vi "(SubVI)Serial_User Code Verification.vi"(8 "에러 입력(에러 없음)":errorcluster, 10 "Data to Write":u8[](array[numeric]), 11 "Read Data":u8[](array[numeric])) -> (0 "에러 출력":errorcluster, 3 "Read Data":u8[](array[numeric]))   [LabVIEW 2020]
panel:
  # "(SubVI)Serial_User Code Verification.vi By hspark\n\nDescription : 시리얼 통신 Write-Read 동작 시 프로토콜 중 Header(6Byte) 다음 2Byte에 대해 검증하는 VI\n                   쓰기한 데이터와 읽기한 데이터가 같은 경우 pass. 다를 경우 에러 발생시킴\n\nInput : \n1. Read Data : 시리얼 통신으로 읽은 데이터 입력\n2. Data to Write : 시리얼 통신으로 쓴 데이터 입력\n\nOutput : \n1. Read Data : Read Data 입력 중 검증한 2Byte를 제외한 나머지 데이터 출력\n\nLabVIEW Version : 2020 SP1 이상\n\nNote : 에러 발생 시 에러 코드는 부여하지 않음. 필요 시 사용자 에러 코드 부여할 것.\n\nUpdate : 2021.10.06"
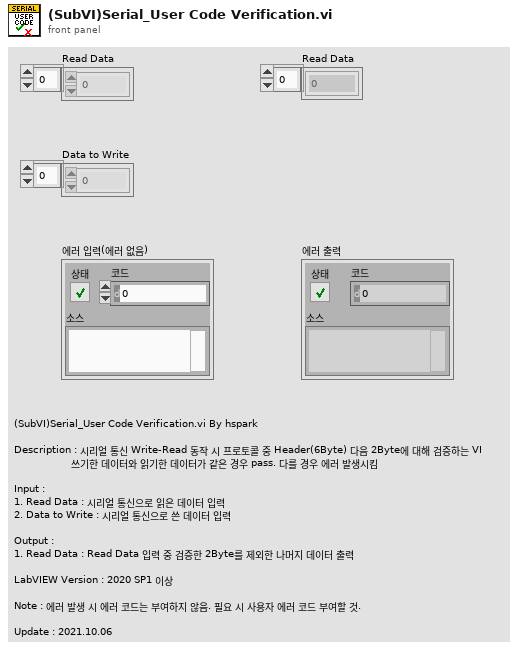
[diagram p1: front panel]
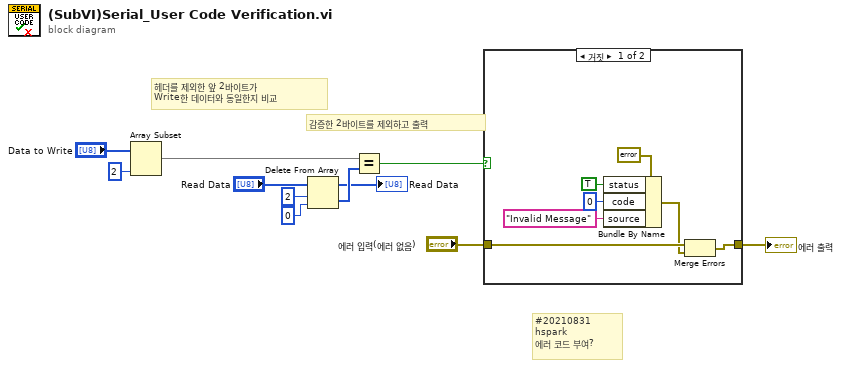
[diagram p0: block diagram]
diagram:
  # "감증한 2바이트를 제외하고 출력"
  # "헤더를 제외한 앞 2바이트가\nWrite한 데이터와 동일한지 비교"
  # "#20210831\nhspark\n에러 코드 부여?"
  n1 = Array Subset(array="Data to Write", length=2 ("길이(나머지)")) -> (w8:u8[])  [unwired: 1 in]
  n2 = Delete From Array(array="Read Data", length=2 ("길이(나머지)"), index=0 ("인덱스")) -> (deleted portion=w2:u8[], array with subset deleted=→"Read Data":u8[])
  n3 = Equal?(x=w8, y=w2) -> (x = y?=w9:bool)
  n4 = case shown="거짓" w9 {
    tunnel: "에러 입력(에러 없음)" -> [w14 w19]
    tunnel: [w13 w19] -> w11
    frame False {
      n5 = Bundle By Name(cluster=errorcluster {"status"=FALSE, "code"=0, "source"=""} ("error out"), "status"=TRUE, "code"=0, "source"="Invalid Message" ("문자열")) -> (w12:errorcluster)
      n6 = Merge Errors(w14, w12) -> (w13:errorcluster)
    }
    frame True {
    }
  }
  "에러 출력" <- w11
